vi "upgrade_line.vi"(0 "Lines":string, 2 "Fault line":string="52-53") -> (6 "Update lines":string, 7 "ñ encontrado?":bool, 8 "From":i32, 9 "To":i32)   [LabVIEW 2020]
panel:
  out "match substring":string
  # "INSERE NÓ VIRTUAL"
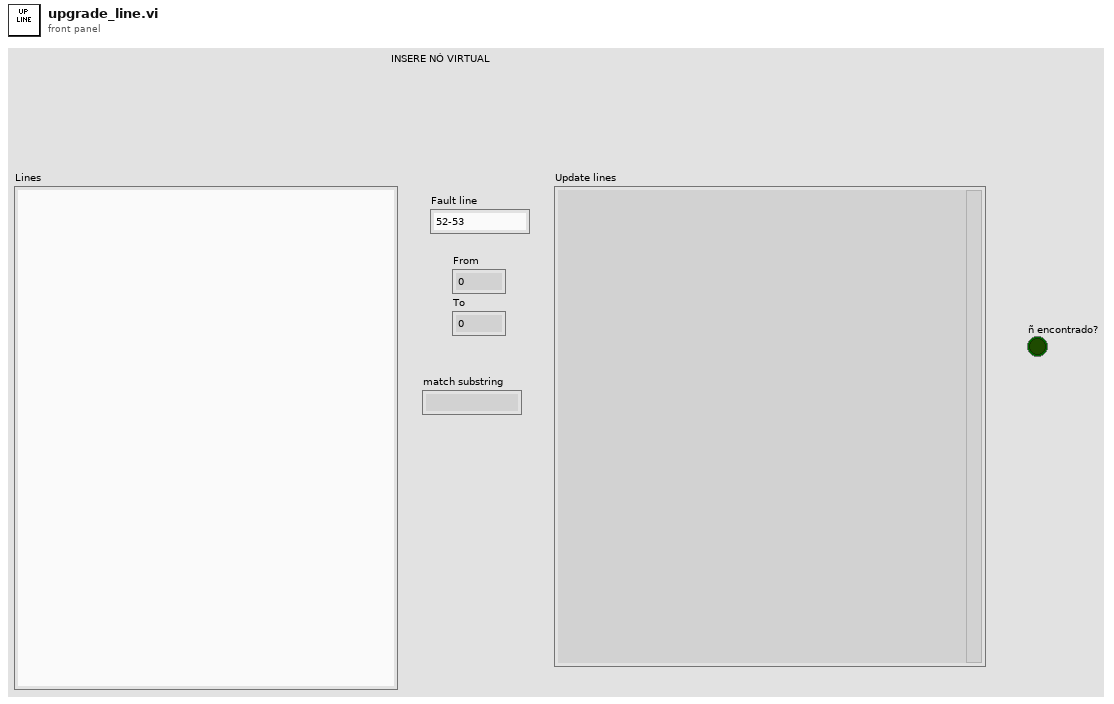
[diagram p1: front panel]
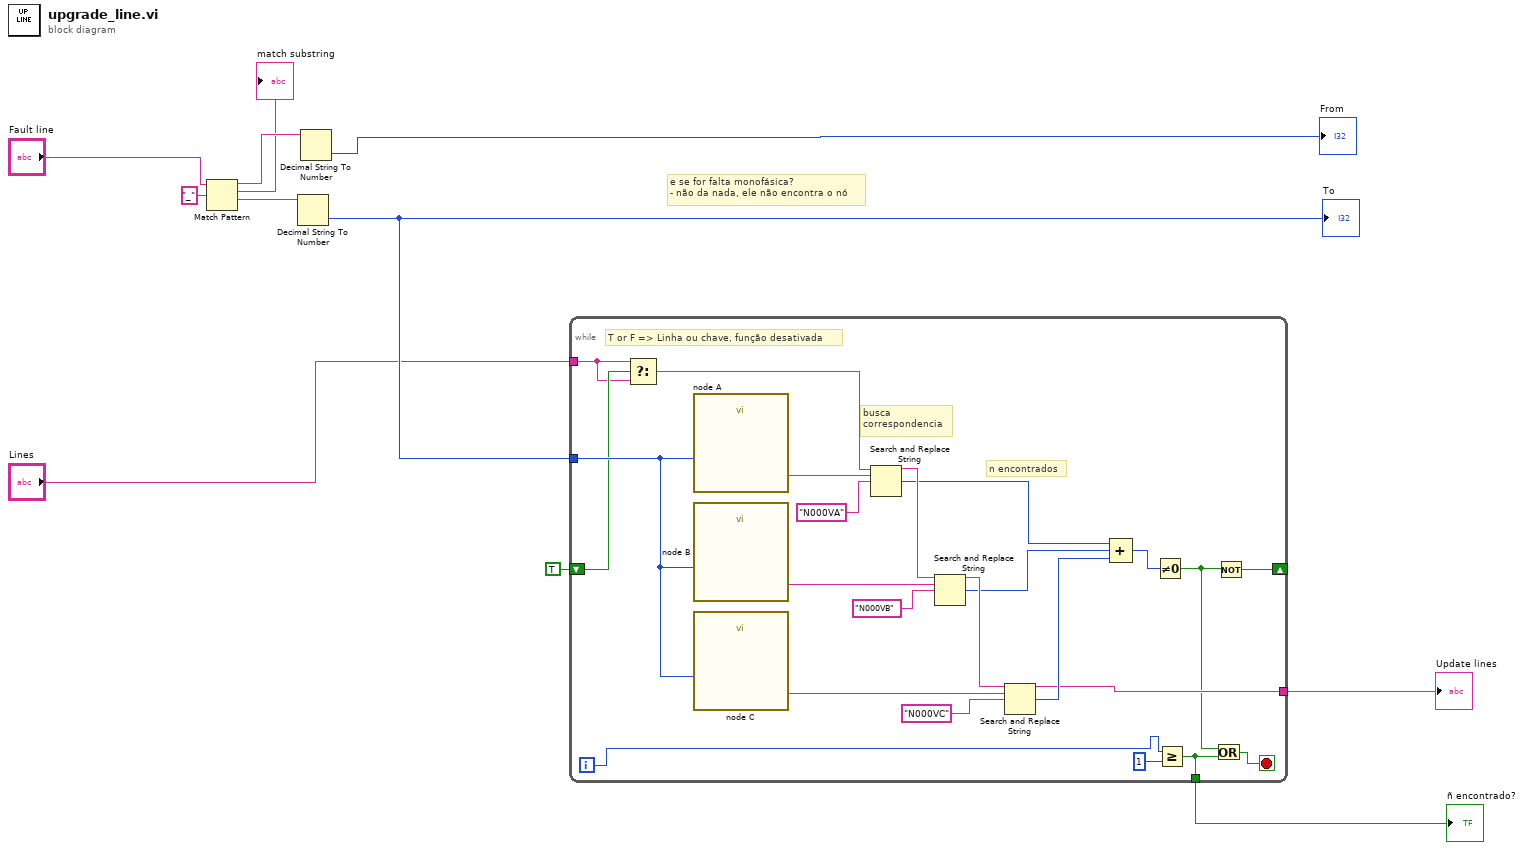
[diagram p0: block diagram]
diagram:
  # "e se for falta monofásica?\n- não da nada, ele não encontra o nó"
  n1 = Match Pattern(string="Fault line", regular expression="_") -> (before substring=w9:string, match substring=→"match substring":string, after substring=w8:string)  [unwired: 1 in, 1 out]
  n2 = Decimal String To Number(string=w8) -> (number=w5:i32)  [unwired: 2 in, 1 out]
  "To" <- w5
  n3 = Decimal String To Number(string=w9) -> (number=→"From":i32)  [unwired: 2 in, 1 out]
  n4 = while {
    tunnel: w5 -> [w33]
    tunnel: "Lines" -> [w12]
    shift-right: [w21] -> _
    shift-left: TRUE -> [w20]
    tunnel: [w19] -> w6
    tunnel: [w13] -> w4
    i -> [w17]
    stop <- w15 stop-if-true
    # "T or F => Linha ou chave, função desativada"
    # "n encontrados"
    # "busca\ncorrespondencia"
    n5 = Select(t=w12, s=w20, f=w12) -> (s? t:f=w25:string)
    n6 = call "node A"("node"=w33) -> ("Result"=w32:string)  [unwired: 13 in, 1 out]
    n7 = call "node B"("node"=w33) -> ("Result"=w31:string)  [unwired: 13 in, 1 out]
    n8 = call "node C"("node"=w33) -> ("Result"=w27:string)  [unwired: 13 in, 1 out]
    n9 = Search and Replace String(input string=w25, search string=w32, replace string="N000VA" ("replace string (\"\")")) -> (result string=w30:string, number of replacements=w22:i32)  [unwired: 5 in, 2 out]
    n10 = Search and Replace String(input string=w30, search string=w31, replace string="N000VB" ("replace string (\"\")")) -> (result string=w28:string, number of replacements=w23:i32)  [unwired: 5 in, 2 out]
    n11 = Search and Replace String(input string=w28, search string=w27, replace string="N000VC" ("replace string (\"\")")) -> (result string=w19:string, number of replacements=w24:i32)  [unwired: 5 in, 2 out]
    n12 = Compound Arithmetic op=ADD(w22, w23, w24) -> (w18:i32)
    n13 = Not Equal To 0?(x=w18) -> (x != 0?=w14:bool)
    n14 = Greater Or Equal?(x=w17, y=1) -> (x >= y?=w13:bool)
    n15 = Or(x=w14, y=w13) -> (x .or. y?=w15:bool)
    n16 = Not(x=w14) -> (.not. x?=w21:bool)
  }
  "Update lines" <- w6
  "ñ encontrado?" <- w4
